vi "Ex2.vi"() -> ()   [LabVIEW 2017]
panel:
  out "?":u8(slide) scale=0.0..100.0
  in  "Soupape":bool
  out "Citerne":dbl(slide) scale=0.0..100.0
  out "Résevoir":dbl(slide) scale=0.0..100.0
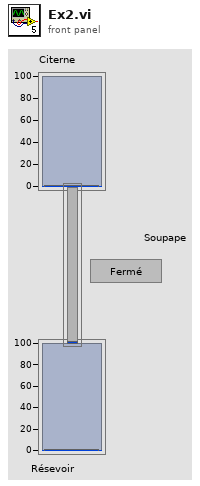
[diagram p1: front panel]
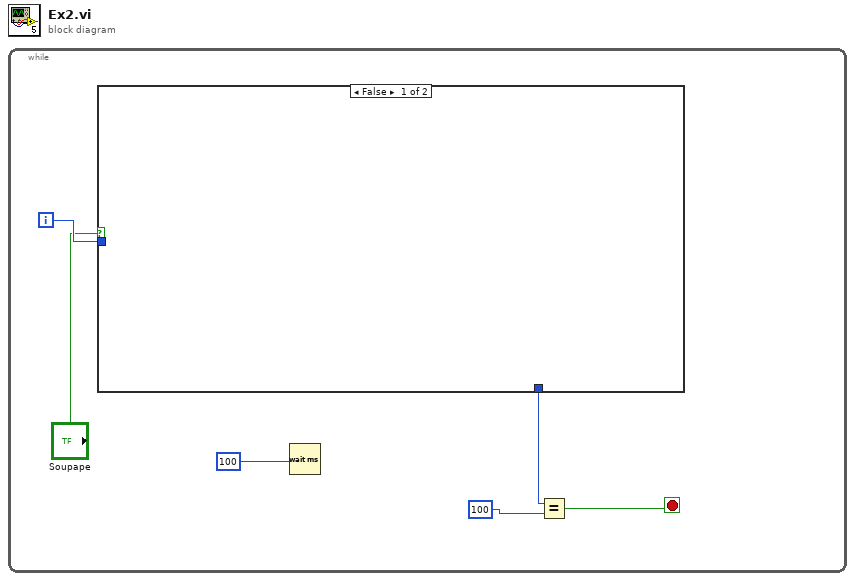
[diagram p0: block diagram]
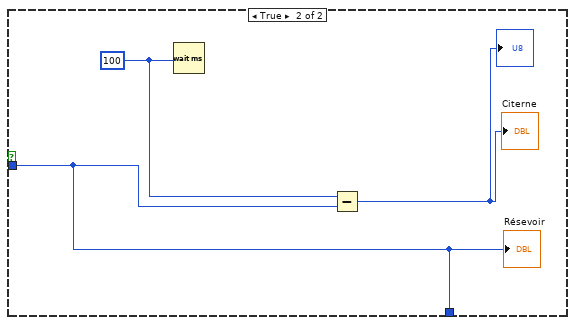
[diagram p2: hidden frame]
diagram:
  n1 = while {
    i -> [w6]
    stop <- w4 stop-if-true
    n2 = case shown="False" "Soupape" {
      tunnel: w6 -> [_ w7]
      tunnel: [_ w7] -> w1
      frame False {
      }
      frame True {
        w9 = 100
        n3 = Wait (ms)(milliseconds to wait=w9) -> ()  [unwired: 1 out]
        n4 = Subtract(x=w9, y=w7) -> (x-y=→"Citerne" →"?":i32)
        "Résevoir" <- w7
      }
    }
    n5 = Wait (ms)(milliseconds to wait=100) -> ()  [unwired: 1 out]
    n6 = Equal?(x=w1, y=100) -> (x = y?=w4:bool)
  }
